vi "Decode Topic Subscriptions.vi"(10 "Payload":u8[](array[numeric]) format="%08b") -> (1 "Valid?":bool, 2 "Topic Subscriptions":string[](array[string]))   [LabVIEW 2013, in "MQTT_Control_Packets.lvlib" / "UNSUBSCRIBE.lvclass"]
uses:
  UNSUBSCRIBE.lvclass
  ControlPacket/ControlPacket.lvclass
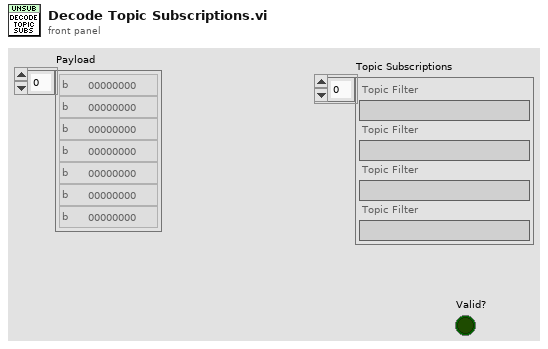
[diagram p1: front panel]
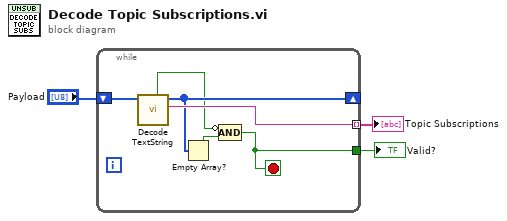
[diagram p0: block diagram]
diagram:
  n1 = while {
    shift-right: [w7] -> _
    shift-left: "Payload" -> [w9]
    tunnel: [w8] -> w1 mode=indexing
    tunnel: [w4] -> w3
    stop <- w4 stop-if-true
    n2 = call "Decode TextString.vi"("Length-Prefixed Field"=w9) -> ("Text String"=w8:string, "Remaining Packets"=w7:u8[], "restricted code"=w6:bool)  [unwired: 8 in]
    n3 = Empty Array?(array=w7) -> (empty?=w5:bool)
    n4 = Compound Arithmetic op=AND(invert w6, w5) -> (w4:bool)
  }
  "Valid?" <- w3
  "Topic Subscriptions" <- w1
